vi "Configure Output.vi"(6 "Enable Output (T: Enable)":bool=TRUE, 7 "Channel (1:CH1)":u16(ring)=1 items=["CH1"=1, "CH2"=2], 8 "error in (no error)":errorcluster, 9 "Current (0 A)":dbl min=0.0 max=3.2 format="%.3f", 10 "Voltage (0 V)":dbl min=0.0 max=32.0 format="%.3f", 11 "VISA resource name":refnum<visa-resource-name>) -> (0 "error out":errorcluster, 3 "VISA resource name out":refnum<visa-resource-name>)   [LabVIEW 2015, in "Siglent SPD3000 Series.lvlib"]
doc: "Configures output voltage level, current level, channel, and enables or disables the output of the power supply."
uses:
  <instrlib>/Siglent SPD3000 Series/Siglent SPD3000 Series.lvlib
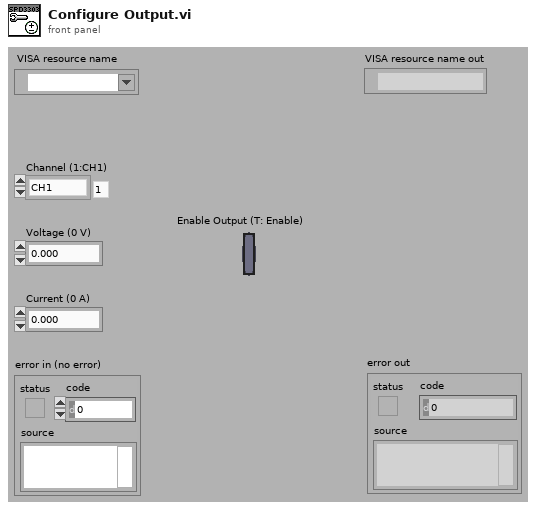
[diagram p1: front panel]
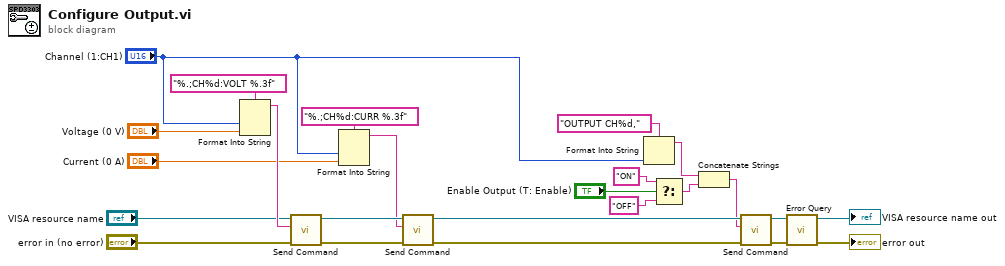
[diagram p0: block diagram]
diagram:
  n1 = Format Into String(format string="%.;CH%d:VOLT %.3f" ("Write buffer"), "Channel (1:CH1)", "Voltage (0 V)") -> (resulting string=w18:string)  [unwired: 2 in, 1 out]
  n2 = call <instrlib>:"Send Command.vi"("error in (no error)"="error in (no error)", "Write Buffer (\"\")"=w18, "VISA resource name"="VISA resource name") -> ("error out"=w23:errorcluster, "VISA resource name out"=w24:refnum<visa-resource-name>)  [unwired: 7 in]
  n3 = Format Into String(format string="%.;CH%d:CURR %.3f" ("Write buffer"), "Channel (1:CH1)", "Current (0 A)") -> (resulting string=w17:string)  [unwired: 2 in, 1 out]
  n4 = call <instrlib>:"Send Command.vi"("error in (no error)"=w23, "Write Buffer (\"\")"=w17, "VISA resource name"=w24) -> ("error out"=w21:errorcluster, "VISA resource name out"=w22:refnum<visa-resource-name>)  [unwired: 7 in]
  n5 = Format Into String(format string="OUTPUT CH%d," ("Write buffer"), "Channel (1:CH1)") -> (resulting string=w15:string)  [unwired: 2 in, 1 out]
  n6 = Select(t="ON" ("Write buffer"), s="Enable Output (T: Enable)", f="OFF" ("Write buffer")) -> (s? t:f=w14:string)
  n7 = Concatenate Strings(w15, w14) -> (w13:string)
  n8 = call <instrlib>:"Send Command.vi"("error in (no error)"=w21, "Write Buffer (\"\")"=w13, "VISA resource name"=w22) -> ("error out"=w9:errorcluster, "VISA resource name out"=w10:refnum<visa-resource-name>)  [unwired: 7 in]
  n9 = call <instrlib>:"Error Query.vi"("error in (no error)"=w9, "VISA resource name"=w10) -> ("error out"=→"error out":errorcluster, "VISA resource name out"=→"VISA resource name out":refnum<visa-resource-name>)  [unwired: 6 in, 2 out]
